vi "finalXi_.vi"(10 "Ramp Pattern":dbl[](array[numeric]), 11 "intraY":dbl) -> (3 "Array":dbl[][](array[numeric]))   [LabVIEW 2013]
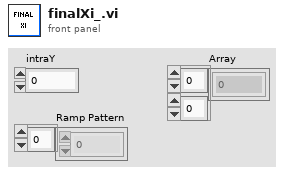
[diagram p1: front panel]
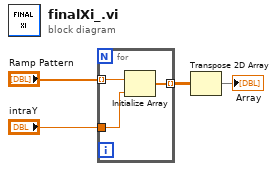
[diagram p0: block diagram]
diagram:
  n1 = for {
    tunnel: "Ramp Pattern" -> [w7] mode=indexing
    tunnel: "intraY" -> [w6]
    tunnel: [w5] -> w2 mode=indexing
    n2 = Initialize Array(w7, w6) -> (w5:dbl[])
  }
  n3 = Transpose 2D Array(2D array=w2) -> (transposed array=→"Array":dbl[][])
